vi "generateSystemMessage.vi"(10 "New Message":string, 11 "Old Message":string) -> (3 "System Message":string)   [LabVIEW 2013]
doc: "Basic Formatting for System Message Box"
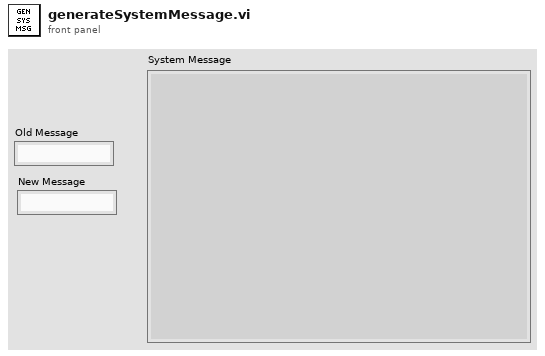
[diagram p1: front panel]
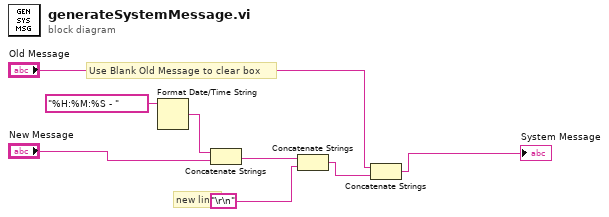
[diagram p0: block diagram]
diagram:
  # "Use Blank Old Message to clear box"
  # "new line"
  n1 = Format Date/Time String(time format string (%c)="%H:%M:%S - ") -> (date/time string=w3:string)  [unwired: 2 in]
  n2 = Concatenate Strings(w3, "New Message") -> (w5:string)
  n3 = Concatenate Strings(w5, "\r\n") -> (w7:string)
  n4 = Concatenate Strings("Old Message", w7) -> (→"System Message":string)
